vi "PmacCommRespStr.vi"(2 "Command String":string, 3 "Device Number i32 (0)":i32 min=0) -> (0 "Response String (\"\")":string, 1 "Response Available Bool (F)":bool)   [LabVIEW 2020]
doc: "Send Command String to PMAC and wait for a response. If Command String is the empty string nothing is sent. Response Available is TRUE when Response String contains response data. When Response Available is FALSE Response String is the empty string. Responses are parsed for PMAC ERR codes and flagged with a modal dialog."
uses:
  Builds/5-8-13/data/PComm32W.dll
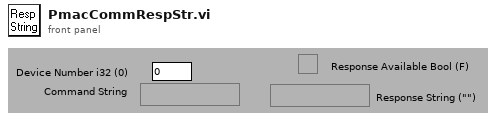
[diagram p1: front panel]
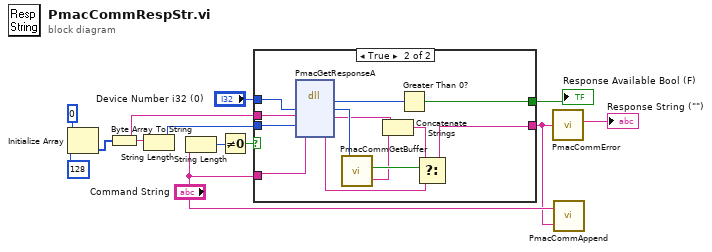
[diagram p0: block diagram]
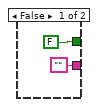
[diagram p2: hidden frame]
diagram:
  n1 = Initialize Array(u8 0, 128) -> (w4:u8[])
  n2 = Byte Array To String(unsigned byte array=w4) -> (string=w2:string)
  n3 = String Length(string=w2) -> (length=w11:i32)
  n4 = String Length(string="Command String") -> (length=w9:i32)
  n5 = Not Equal To 0?(x=w9) -> (x != 0?=w10:bool)
  n6 = case shown="True" w10 {
    tunnel: "Device Number i32 (0)" -> [_ w22]
    tunnel: [FALSE w15] -> w1
    tunnel: w11 -> [_ w24]
    tunnel: "Command String" -> [_ w23]
    tunnel: ["" w20] -> w6
    tunnel: w2 -> [_ w16]
    frame False {
    }
    frame True {
      n7 = dll-call lib="C:/NUWAR_Master/Builds/5-8-13/data/PComm32W.dll" fn="PmacGetResponseA"("DeviceNumber"=w22, "ResponseString"=w16, "MaxStringLength"=w24, "CommandString"=w23) -> ("return type"=w25:i32, "ResponseString"=w18:string)  [unwired: 6 in, 2 out]
      n8 = call "PmacCommGetBuffer.vi"("Device Number i32 (0)"=w22) -> ("Response Available Bool (F)"=w21:bool, "Response String (\"\")"=w17:string)
      n9 = Concatenate Strings(w18, w17) -> (w19:string)
      n10 = Greater Than 0?(x=w25) -> (x > 0?=w15:bool)
      n11 = Select(t=w19, s=w21, f=w18) -> (s? t:f=w20:string)
    }
  }
  "Response Available Bool (F)" <- w1
  n12 = call "PmacCommError.vi"("Input String"=w6) -> ("Output String"=→"Response String (\"\")":string)  [unwired: 3 out]
  n13 = call "PmacCommAppend.vi"("Response String"=w6, "Command String"="Command String") -> ()
